vi "topo_star.vi"(4 "deltat (TT-UT1)":dbl[unit], 5 "TimeStamp [UT1]":timestamp format="%<%H:%M:%S%6u\n%Y/%m/%d>T", 6 "error in (no error)":errorcluster, 7 "on_surface":T2 {"longitude" format="%_10g"; "latitude" format="%_10g"}, 8 "cat_entry":T1 {"dec" format="%.6g"; "ra" format="%.6g"}) -> (0 "error out":errorcluster, 3 "ra/dec":cluster{"ra":dbl[unit], "dec":dbl[unit]} {"dec" format="%_10g"; "ra" format="%_10g"})   [LabVIEW 2009]
uses:
  SiteInformation.ctl
  StarAstrometricEntry.ctl
  lib/novas-dll.dll
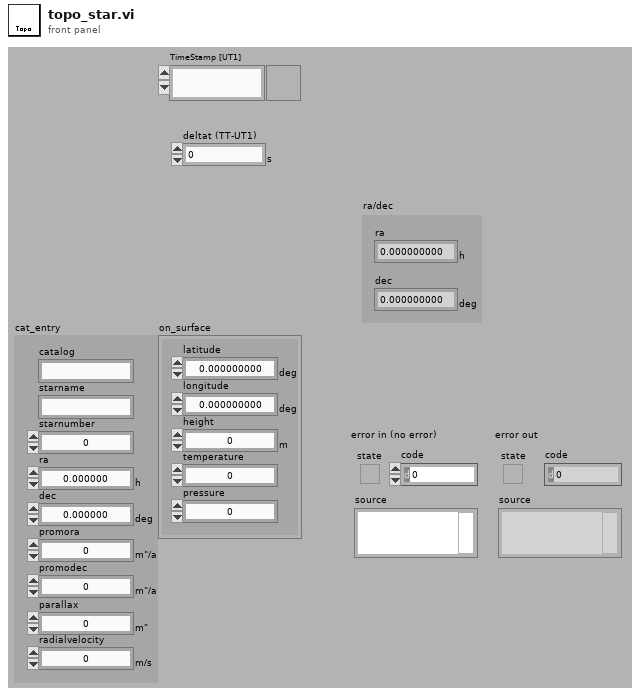
[diagram p1: front panel]
types:
  T1 = typedef "StarAstrometricEntry.ctl" = cluster{"catalog":string, "starname":string, "starnumber":i32, "ra":dbl[unit], "dec":dbl[unit], "promora":dbl[unit], "promodec":dbl[unit], "parallax":dbl[unit], "radialvelocity":dbl[unit]}
  T2 = typedef "SiteInformation.ctl" = cluster{"latitude":dbl[unit], "longitude":dbl[unit], "height":dbl[unit], "temperature":dbl, "pressure":dbl}
  T3 = cluster{"catalog":string, "starname":string, "starnumber":i32, "ra":dbl, "dec":dbl, "promora":dbl, "promodec":dbl, "parallax":dbl, "radialvelocity":dbl}
  T4 = cluster{"latitude":dbl, "longitude":dbl, "height":dbl, "temperature":dbl, "pressure":dbl}
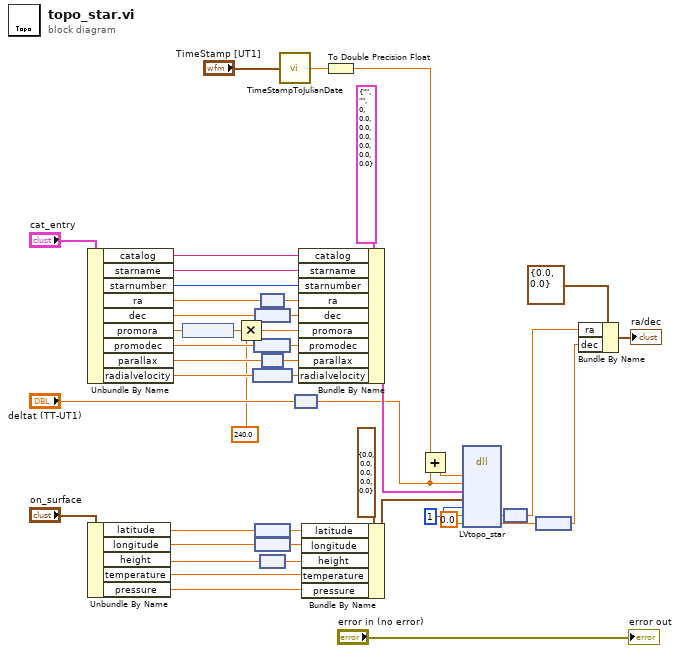
[diagram p0: block diagram]
diagram:
  w44 = 0.0 ("dec")
  n1 = Unbundle By Name("cat_entry") -> ("catalog"=w25:string, "starname"=w24:string, "starnumber"=w23:i32, "ra"=w22:dbl[unit], "dec"=w21:dbl[unit], "promora"=w10:dbl[unit], "promodec"=w20:dbl[unit], "parallax"=w19:dbl[unit], "radialvelocity"=w18:dbl[unit])
  n2 = Unbundle By Name("on_surface") -> ("latitude"=w40:dbl[unit], "longitude"=w39:dbl[unit], "height"=w38:dbl[unit], "temperature"=w37:dbl, "pressure"=w36:dbl)
  n3 = node(w10) -> (w9:dbl)
  n4 = Multiply(x=w9, y=240.0) -> (x*y=w7:dbl)
  n5 = node(w18) -> (w13:dbl)
  n6 = node(w20) -> (w15:dbl)
  n7 = node(w21) -> (w16:dbl)
  n8 = node(w40) -> (w33:dbl)
  n9 = node(w39) -> (w34:dbl)
  n10 = node(w38) -> (w35:dbl)
  n11 = node(w22) -> (w17:dbl)
  n12 = node(w19) -> (w14:dbl)
  n13 = call "TimeStampToJulianDate.vi"("TimeStamp [UT]"="TimeStamp [UT1]") -> ("JulianDay"=w2:ext)
  n14 = node("deltat (TT-UT1)") -> (w4:dbl)
  n15 = Bundle By Name(cluster=T3 {"catalog"="", "starname"="", "starnumber"=0, "ra"=0.0, "dec"=0.0, "promora"=0.0, "promodec"=0.0, "parallax"=0.0, "radialvelocity"=0.0} ("cat_entry"), "catalog"=w25, "starname"=w24, "starnumber"=w23, "ra"=w17, "dec"=w16, "promora"=w7, "promodec"=w15, "parallax"=w14, "radialvelocity"=w13) -> (w28:T3)
  n16 = Bundle By Name(cluster=T4 {"latitude"=0.0, "longitude"=0.0, "height"=0.0, "temperature"=0.0, "pressure"=0.0} ("site_info"), "latitude"=w33, "longitude"=w34, "height"=w35, "temperature"=w37, "pressure"=w36) -> (w41:T4)
  n17 = To Double Precision Float(number=w2) -> (double precision float=w1:dbl)
  n18 = Add(x=w1, y=w4) -> (x+y=w3:dbl)
  n19 = dll-call lib="C:/OhanaOS/Instruments/Novas/lib/novas-dll.dll" fn="LVtopo_star"("jd_tt"=w3, "delta_t"=w4, "star"=w28, "location"=w41, "accuracy"=i8 1, "ra"=w44, "dec"=w44) -> ("ra"=w45:dbl, "dec"=w46:dbl)  [unwired: 5 in, 6 out]
  n20 = node(w45) -> (w30:dbl[unit])
  n21 = node(w46) -> (w29:dbl[unit])
  n22 = Bundle By Name(cluster=cluster{"ra":dbl[unit], "dec":dbl[unit]} {"ra"=0.0, "dec"=0.0} ("ra/dec"), "ra"=w30, "dec"=w29) -> (→"ra/dec":cluster{"ra":dbl[unit], "dec":dbl[unit]})
  "error out" <- "error in (no error)"
